vi "CRYAna Loose Particles.vi"(4 "Loose part":T1, 5 "FStop":dbl=20.0 min=1.0, 6 "Unit Info":T4={"Y unit In"="dB", "dB ref In"=1.0, "Y unit Out"="dB", "dB ref Out"=1.0, "Y unit Curve"="dB", "dB ref Curve"=1.0, "Y data  Curve"=0, "Y data Time"=0}, 7 "FStart":dbl=1000.0 min=1.0, 8 "Fs":dbl=44100.0 min=1.0, 9 "Response":dbl[](array[numeric]), 10 "Stimulus":dbl[](array[numeric]), 11 "Channel Label In":string) -> (2 "Value Out":T3[](array[typedef]) {"Z data" items=["dB", "Lin"]; "X data" items=["dB", "Lin"]; "Y data" items=["dB", "Lin"]; "Z dB ref" format="%.1f"; "Z axis" items=["Log", "Lin"]; "X dB ref" format="%.1f"; "X axis" items=["Log", "Lin"]; "Y axis" items=["Log", "Lin"]; "Y dB ref" format="%.1f"; "Curve"."z" format="%.2f"; "Curve"."y" format="%.2f"; "Curve"."x" format="%.2f"}, 3 "Wave out":T2[](array[typedef]) {"Y dB ref" format="%.1f"; "Y axis" items=["Log", "Lin"]; "Y data" items=["dB", "Lin"]; "X data" items=["dB", "Lin"]})   [LabVIEW 2013]
uses:
  Typedef Control/CRYWaveform Cluster.ctl
  Typedef Control/CRYUnit Info Cluster.ctl
  Typedef Control/CRYData Cluster.ctl
  Typedef Control/CRYStimulus Test Infor Cluster.ctl
panel:
  in  "Waveform Cluster Out":T2={"Waveform"={"X0"=0.0, "dX"=0.0, "Y"=[]}, "X data"=1, "Y data"=0, "Y axis"=0, "X unit"="s", "Y unit"="", "Y dB ref"=1.0, "display Y"=TRUE, "display X"=FALSE, "Overload?"=FALSE, "Test Info"="", "Step No."=0, "Name"="", "protected"=FALSE, "Sqc history"=[], "Signal Channel ID"=0, "Plot Settings"={"Color"=0, "Interpolation"=0, "Point Style"=0, "Line Style"=0, "Point Color"=0, "Line Width"=0, "Bar Plot Style"=0, "Fill To"=0}, "AutoProtect"=FALSE} {"Y dB ref" format="%.1f"; "Y axis" items=["Log", "Lin"]; "Y data" items=["dB", "Lin"]; "X data" items=["dB", "Lin"]}
  in  "Infor":T5 {"Sens In" format="%.2f"}
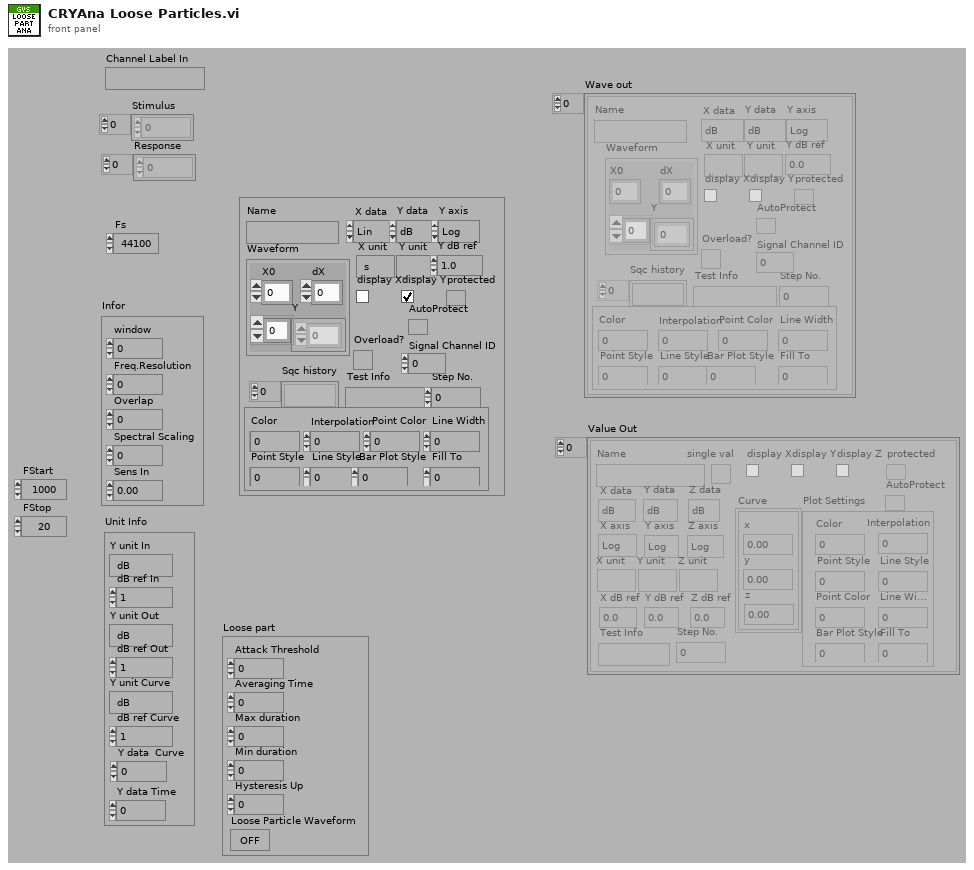
[diagram p1: front panel]
types:
  T1 = cluster{"Attack Threshold":dbl, "Averaging Time":dbl, "Max duration":dbl, "Min duration":dbl, "Hysteresis Up":dbl, "Loose Particle Waveform":bool}
  T2 = typedef "CRYWaveform Cluster.ctl" = cluster{"Waveform":cluster{"X0":dbl, "dX":dbl, "Y":sgl[]}, "X data":u16, "Y data":u16, "Y axis":u16, "X unit":string, "Y unit":string, "Y dB ref":dbl, "display Y":bool, "display X":bool, "Overload?":bool, "Test Info":string, "Step No.":i32, "Name":string, "protected":bool, "Sqc history":string[], "Signal Channel ID":i32, "Plot Settings":cluster{"Color":u32, "Interpolation":u8, "Point Style":u8, "Line Style":u8, "Point Color":u32, "Line Width":u8, "Bar Plot Style":u8, "Fill To":i16}, "AutoProtect":bool}
  T3 = typedef "CRYData Cluster.ctl" = cluster{"Name":string, "Curve":cluster{"x":dbl, "y":dbl, "z":dbl}[], "X data":u16, "Y data":u16, "Z data":u16, "X axis":u16, "Y axis":u16, "Z axis":u16, "X unit":string, "Y unit":string, "Z unit":string, "X dB ref":dbl, "Y dB ref":dbl, "Z dB ref":dbl, "single val":bool, "protected":bool, "display X":bool, "display Y":bool, "display Z":bool, "Test Info":string, "Step No.":i32, "Plot Settings":cluster{"Color":u32, "Interpolation":u8, "Point Style":u8, "Line Style":u8, "Point Color":u32, "Line Width":u8, "Bar Plot Style":u8, "Fill To":i16}, "AutoProtect":bool}
  T4 = typedef "CRYUnit Info Cluster.ctl" = cluster{"Y unit In":string, "dB ref In":dbl, "Y unit Out":string, "dB ref Out":dbl, "Y unit Curve":string, "dB ref Curve":dbl, "Y data  Curve":u16, "Y data Time":u16}
  T5 = cluster{"window":u16, "Freq.Resolution":dbl, "Overlap":dbl, "Spectral Scaling":u16, "Sens In":dbl}
  T6 = typedef "CRYStimulus Test Infor Cluster.ctl" = cluster{"Stimulus Type":string, "Signal Type":string, "In/Out":bool, "FAPS":cluster{"freq":dbl, "ampl":dbl, "cycles":dbl, "samples":i32}[], "Sampling Rate":dbl, "Samples":i32, "Analysis Param":string, "Resolution":u16, "Steps":u32, "Analysis Value":dbl[], "Diff Freq":dbl, "FStart":dbl, "FStop":dbl, "Calibration Param":string, "Anti Alias":dbl, "Level Out1":dbl, "Level Out2":dbl, "EQ":bool}
  T7 = cluster{"display X":bool, "display Y":bool, "display Z":bool}[]
  T8 = cluster{"X unit":string, "X data":u16, "Y unit":string, "Y data Time":u16, "Z unit":string, "X data":u16, "dB ref":dbl}[]
  T9 = typedef "CRYUnit Info Out Cluster.ctl" = cluster{"X unit":string, "X data":u16, "Y unit":string, "Y data Time":u16, "Z unit":string, "X axis":u16, "X dB ref":dbl, "Y dB ref":dbl, "single/curve":bool}
  T10 = typedef "CRYAnalysis CurveName Cluster.ctl" = cluster{"Custom Curve Name":string, "Custom Curve ID":i32, "Default Curve Name":string}[]
  T11 = cluster{"X unit":string, "X data":u16, "Y unit":string, "Y data Time":u16, "Z unit":string, "X data":u16, "dB ref":dbl}
  T12 = cluster{"display X":bool, "display Y":bool, "display Z":bool}
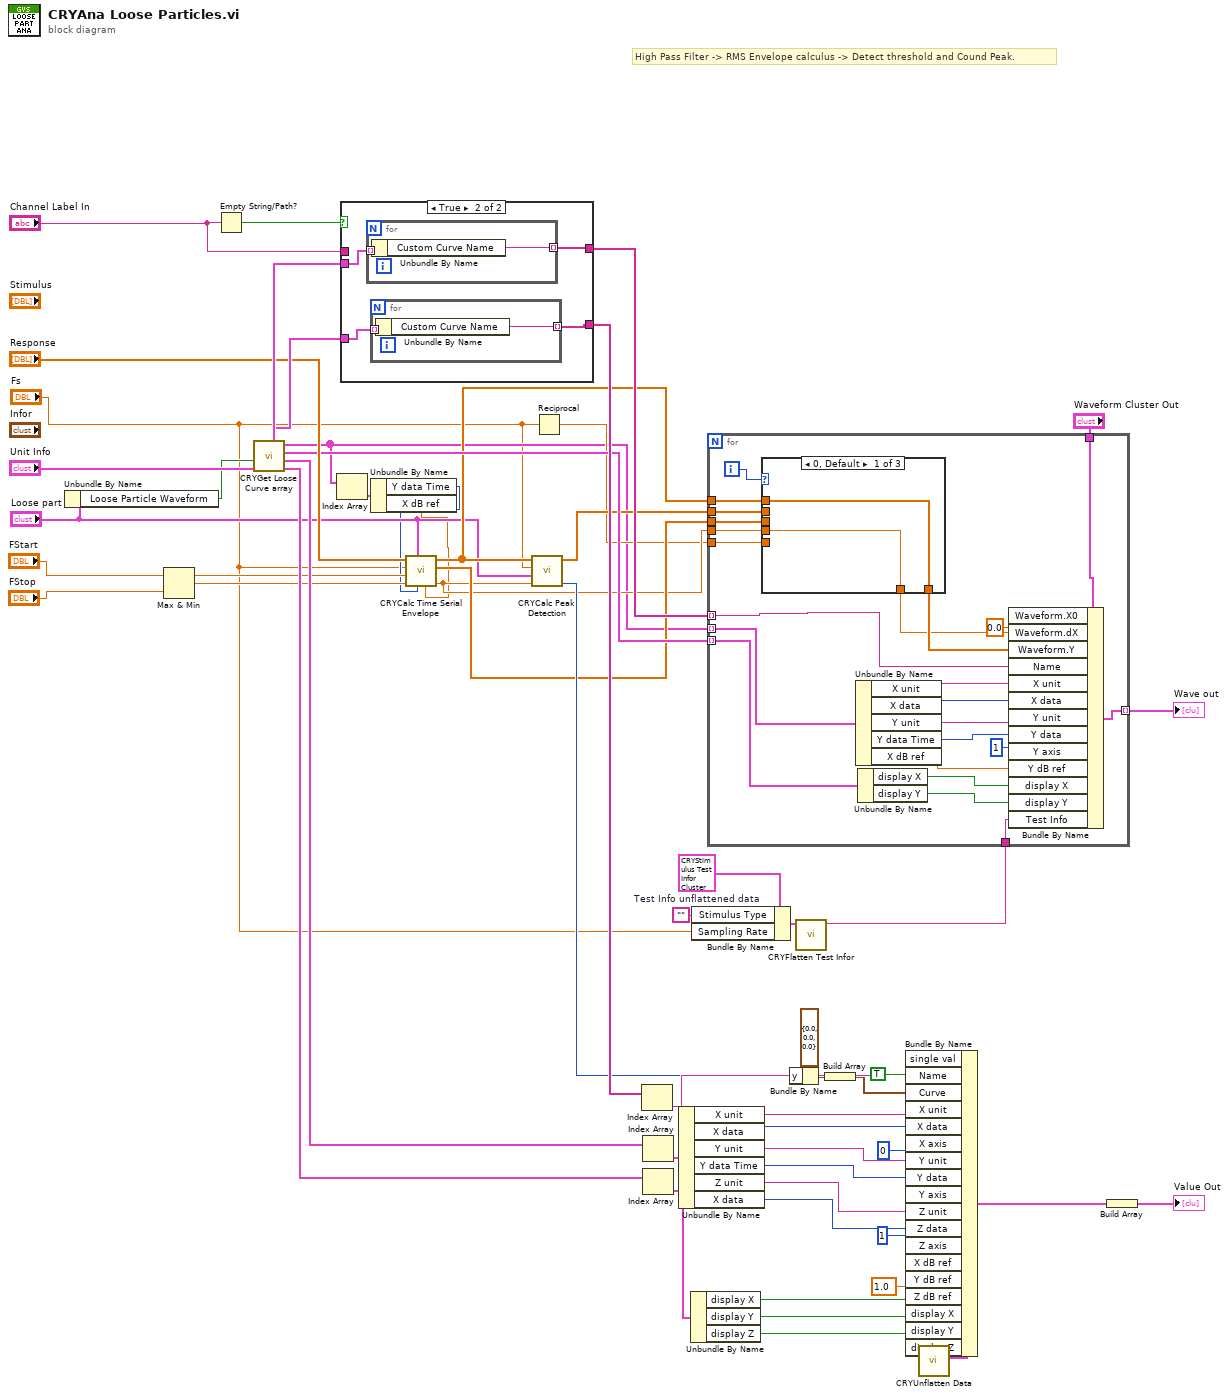
[diagram p0: block diagram]
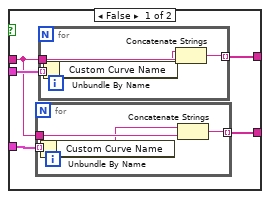
[diagram p4: hidden frame]
diagram:
  w3 = T6 {"Stimulus Type"="", "Signal Type"="", "In/Out"=FALSE, "FAPS"=[], "Sampling Rate"=0.0, "Samples"=0, "Analysis Param"="", "Resolution"=0, "Steps"=0, "Analysis Value"=[], "Diff Freq"=0.0, "FStart"=0.0, "FStop"=0.0, "Calibration Param"="", "Anti Alias"=0.0, "Level Out1"=0.0, "Level Out2"=0.0, "EQ"=FALSE}  # Test Info unflattened data
  w47 = 1.0 ("X dB ref")
  w46 = u16 1 ("Y data")
  # "High Pass Filter -> RMS Envelope calculus -> Detect threshold and Cound Peak."
  n1 = Unbundle By Name("Loose part") -> ("Loose Particle Waveform"=w10:bool)
  n2 = Max & Min(x="FStart", y="FStop") -> (max(x,y)=w23:dbl, min(x,y)=w22:dbl)
  n3 = Empty String/Path?(string/path="Channel Label In") -> (empty?=w53:bool)
  n4 = call "CRYGet Loose Curve array.vi"("Unit Info In"="Unit Info", "Loose Particle Waveform"=w10) -> ("Value Display Array"=w55:T7, "Value Unit Info Out"=w54:T8, "WMF Display Array"=w20:T7, "WFM Unit Info Out"=w9:T9[], "Curve Info Array Out"=w31:T10, "WFM Info Array Out"=w52:T10)  [unwired: 4 in]
  n5 = Index Array(array=w9) -> (element=w8:T9)  [unwired: 1 in]
  n6 = case shown="True" w53 {
    tunnel: w52 -> [w61 w73]
    tunnel: "Channel Label In" -> [w58 _]
    tunnel: [w60 w71] -> w17
    tunnel: w31 -> [w59 w72]
    tunnel: [w57 w70] -> w30
    frame False {
      n7 = for {
        tunnel: w59 -> [w63] mode=indexing
        tunnel: w58 -> [w65]
        tunnel: [w64] -> w57 mode=indexing
        n8 = Unbundle By Name(w63) -> ("Custom Curve Name"=w62:string)
        n9 = Concatenate Strings(w62, w65) -> (w64:string)
      }
      n10 = for {
        tunnel: w61 -> [w67] mode=indexing
        tunnel: w58 -> [w69]
        tunnel: [w68] -> w60 mode=indexing
        n11 = Unbundle By Name(w67) -> ("Custom Curve Name"=w66:string)
        n12 = Concatenate Strings(w66, w69) -> (w68:string)
      }
    }
    frame True {
      n13 = for {
        tunnel: w73 -> [w77] mode=indexing
        tunnel: [w76] -> w71 mode=indexing
        n14 = Unbundle By Name(w77) -> ("Custom Curve Name"=w76:string)
      }
      n15 = for {
        tunnel: w72 -> [w75] mode=indexing
        tunnel: [w74] -> w70 mode=indexing
        n16 = Unbundle By Name(w75) -> ("Custom Curve Name"=w74:string)
      }
    }
  }
  n17 = Unbundle By Name(w8) -> ("Y data Time"=w7:u16, "X dB ref"=w6:dbl)
  n18 = call "CRYCalc Time Serial Envelope.vi"("dB ref"=w6, "Y data"=w7, "Loose part Info"="Loose part", "FStop"=w22, "FStart"=w23, "Fs"="Fs", "Signal In"="Response") -> ("Loose Particle dT"=w13:dbl, "Loose Particle Wave Out"=w14:dbl[], "Loose Particle Envelope Out"=w16:dbl[])  [unwired: 2 in]
  n19 = call "CRYCalc Peak Detection.vi"("Loose Particle dT"=w13, "Loose part Info"="Loose part", "Fs"="Fs", "Loose Particle Envelope In"=w16) -> ("number of peaks"=w21:i32, "Loose Particle Threshold"=w15:dbl[])  [unwired: 6 in]
  n20 = Reciprocal(x="Fs") -> (1/x=w12:dbl)
  n21 = Index Array(array=w30) -> (element=w35:string)  [unwired: 1 in]
  n22 = Index Array(array=w54) -> (element=w33:T11)  [unwired: 1 in]
  n23 = Index Array(array=w55) -> (element=w34:T12)  [unwired: 1 in]
  n24 = Unbundle By Name(w33) -> ("X unit"=w43:string, "X data"=w44:u16, "Y unit"=w42:string, "Y data Time"=w41:u16, "Z unit"=w40:string, "X data"=w39:u16)
  n25 = Unbundle By Name(w34) -> ("display X"=w50:bool, "display Y"=w49:bool, "display Z"=w48:bool)
  n26 = Bundle By Name(cluster=w3, "Stimulus Type"="", "Sampling Rate"="Fs") -> (w5:T6)
  n27 = Bundle By Name(cluster=cluster{"x":dbl, "y":dbl, "z":dbl} {"x"=0.0, "y"=0.0, "z"=0.0}, "y"=w21) -> (w28:cluster{"x":dbl, "y":dbl, "z":dbl})
  n28 = call "CRYFlatten Test Infor.vi"("Test Infor data"=w5) -> ("Fattened Data"=w2:string)  [unwired: 10 out]
  n29 = for {
    tunnel: w20 -> [w92] mode=indexing
    tunnel: w9 -> [w91] mode=indexing
    tunnel: [w90] -> w18 mode=indexing
    tunnel: "Waveform Cluster Out" -> [w89]
    tunnel: w17 -> [w79] mode=indexing
    tunnel: w12 -> [w82]
    tunnel: w16 -> [w87]
    tunnel: w15 -> [w85]
    tunnel: w14 -> [w84]
    tunnel: w13 -> [w83]
    tunnel: w2 -> [w78]
    i -> [w88]
    n30 = case shown="0, Default" w88 {
      tunnel: w87 -> [w102 _ _]
      tunnel: [w102 w104 w106] -> w86
      tunnel: w85 -> [_ w104 _]
      tunnel: w84 -> [_ _ w106]
      tunnel: w83 -> [w101 w103 _]
      tunnel: [w101 w103 w105] -> w81
      tunnel: w82 -> [_ _ w105]
      frame 0, Default {
      }
      frame 1 {
      }
      frame 2 {
      }
    }
    n31 = Unbundle By Name(w91) -> ("X unit"=w97:string, "X data"=w93:u16, "Y unit"=w98:string, "Y data Time"=w94:u16, "X dB ref"=w99:dbl)
    n32 = Unbundle By Name(w92) -> ("display X"=w95:bool, "display Y"=w96:bool)
    n33 = Bundle By Name(cluster=w89, "Waveform.X0"=0.0, "Waveform.dX"=w81, "Waveform.Y"=w86, "Name"=w79, "X unit"=w97, "X data"=w93, "Y unit"=w98, "Y data"=w94, "Y axis"=u16 1, "Y dB ref"=w99, "display X"=w95, "display Y"=w96, "Test Info"=w78) -> (w90:T2)
  }
  "Wave out" <- w18
  n34 = Build Array(w28) -> (w27:cluster{"x":dbl, "y":dbl, "z":dbl}[])
  n35 = call "CRYUnflatten Data.vi"() -> ("Datum"=w38:T3)  [unwired: 1 in, 10 out]
  n36 = Bundle By Name(cluster=w38, "single val"=TRUE, "Name"=w35, "Curve"=w27, "X unit"=w43, "X data"=w44, "X axis"=u16 0 ("X data"), "Y unit"=w42, "Y data"=w41, "Y axis"=w46, "Z unit"=w40, "Z data"=w39, "Z axis"=w46, "X dB ref"=w47, "Y dB ref"=w47, "Z dB ref"=w47, "display X"=w50, "display Y"=w49, "display Z"=w48) -> (w36:T3)
  n37 = Build Array(w36) -> (→"Value Out":T3[])
